vi "No_COM_port_found_EXIT.vi"(10 "error in (no error)":errorcluster, 11 "Message In":string) -> (0 "STOP":bool, 1 "Number of COM ports":u32, 2 "Message Out":string, 3 "COM PORTS":string[](array[string]), 5 "error out":errorcluster)   [LabVIEW 2012]
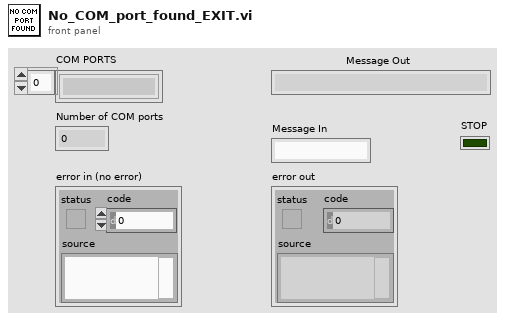
[diagram p1: front panel]
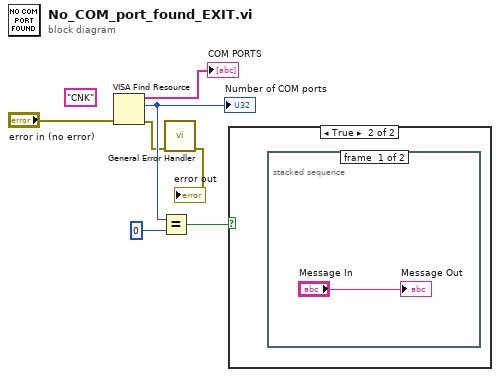
[diagram p0: block diagram]
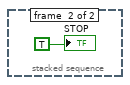
[diagram p3: hidden frame]
diagram:
  (unwired) "CNK"
  n1 = VISA Find Resource(8:"error in (no error)") -> (0:w3:errorcluster, 2:w5:u32, 3:→"COM PORTS":string[])  [unwired: 2 in]
  "Number of COM ports" <- w5
  n2 = Equal?(x=w5, y=0) -> (x = y?=w6:bool)
  n3 = call <vilib>:"General Error Handler.vi"("error in (no error)"=w3) -> ("error out"=→"error out":errorcluster)  [unwired: 1 in, 13 out]
  n4 = case shown="True" w6 {
    frame False {
    }
    frame True {
      n5 = stacked-sequence {
        frame #0 {
          "Message Out" <- "Message In"
        }
        frame #1 {
          "STOP" <- TRUE
        }
      }
    }
  }
